vi "TDT-Initialize.vi"() -> (4 "Server IP Address":u32=4925, 6 "TCP Port":u16=4925, 14 "Data":T1={"TTankX"=refnum, "TDevAccX"=refnum, "LastTime"=0.0, "error"={"status"=FALSE, "code"=0, "source"=""}, "Block Name"="", "Circuit Tag"="", "Tank Name"="", "NumTicks"=0, "LastTick"=0.0, "Idle?"=FALSE, "Wait (ms)"=1000, "LastArtf"=0.0, "LastTosc"=0.0}, 15 "error out":errorcluster)   [LabVIEW 2015]
uses:
  TDT Interface Data.ctl
  <vilib>/Utility/config.llb/Read Key (String).vi
  <vilib>/Utility/config.llb/Read Key (I32).vi
  <vilib>/Utility/config.llb/Read Key (Boolean).vi
  <vilib>/Utility/config.llb/NI_LVConfig.lvlib
panel:
  in  "error in (no error)":errorcluster
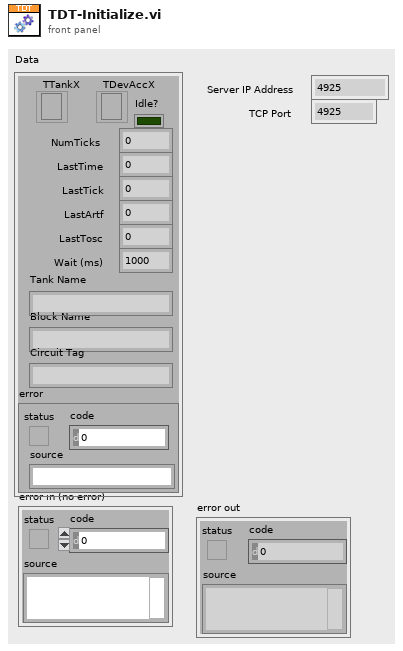
[diagram p1: front panel]
types:
  T1 = typedef "TDT Interface Data.ctl" = cluster{"TTankX":refnum<k7>, "TDevAccX":refnum<k7>, "LastTime":dbl, "error":errorcluster, "Block Name":string, "Circuit Tag":string, "Tank Name":string, "NumTicks":i32, "LastTick":dbl, "Idle?":bool, "Wait (ms)":u32, "LastArtf":dbl, "LastTosc":dbl}
  T2 = typedef "NI_LVConfig.lvlib/Config Data RefNum.ctl" = refnum<k1>
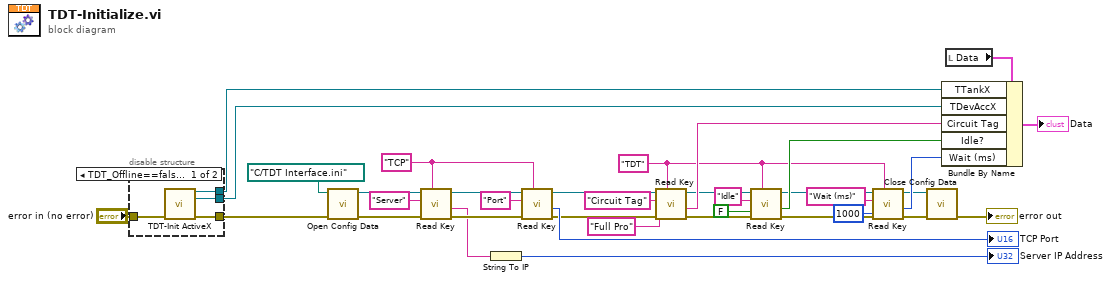
[diagram p0: block diagram]
diagram:
  w2 = "TDT" ("section")
  w29 = "TCP" ("section")
  n1 = disable-structure shown="TDT_Offline==false, Default" {
    disable-tunnel: "error in (no error)" -> [w40 _]
    disable-tunnel: [w39 _] -> w21
    disable-tunnel: [w38 _] -> w20
    disable-tunnel: [w37 _] -> w19
    frame condition #0 (active) {
      n2 = call "TDT-Init ActiveX.vi"("error in (no error)"=w40) -> ("TTANKXLib.TTankX"=w39:refnum<k7>, "TDEVACCXLib.TDevAccX"=w38:refnum<k7>, "error out"=w37:errorcluster)  [unwired: 12 in]
    }
    frame condition #1 {
    }
  }
  n3 = call <vilib>:"Open Config Data.vi"("error in (no error)"=w19, "configuration file path"=path "C:/TDT Interface.ini") -> ("error out"=w33:errorcluster, "refnum"=w34:T2)  [unwired: 7 in, 1 out]
  n4 = call-poly <vilib>:"Read Key.vi"("section"=w29, "error in (no error)"=w33, "key"="Server", "refnum"=w34) -> ("error out"=w31:errorcluster, "value"=w27:string, "refnum out"=w30:T2)  [unwired: 4 in, 1 out]
  n5 = String To IP(1:w27) -> (0:→"Server IP Address":u32)
  n6 = call-poly <vilib>:"Read Key.vi"("section"=w29, "error in (no error)"=w31, "key"="Port", "refnum"=w30) -> ("error out"=w17:errorcluster, "value"=→"TCP Port":i32, "refnum out"=w18:T2)  [unwired: 4 in, 1 out]
  n7 = call-poly <vilib>:"Read Key.vi"("section"=w2, "error in (no error)"=w17, "default value"="Full Pro", "key"="Circuit Tag", "refnum"=w18) -> ("error out"=w12:errorcluster, "value"=w14:string, "refnum out"=w11:T2)  [unwired: 3 in, 1 out]
  n8 = call-poly <vilib>:"Read Key.vi"("section"=w2, "error in (no error)"=w12, "default value"=FALSE, "key"="Idle", "refnum"=w11) -> ("error out"=w7:errorcluster, "value"=w9:bool, "refnum out"=w3:T2)  [unwired: 3 in, 1 out]
  n9 = call-poly <vilib>:"Read Key.vi"("section"=w2, "error in (no error)"=w7, "default value"=1000, "key"="Wait (ms)", "refnum"=w3) -> ("error out"=w6:errorcluster, "value"=w4:i32, "refnum out"=w1:T2)  [unwired: 3 in, 1 out]
  n10 = call <vilib>:"Close Config Data.vi"("error in (no error)"=w6, "refnum"=w1) -> ("error out"=→"error out":errorcluster)  [unwired: 8 in, 1 out]
  n11 = local read "Data"() -> (w22:T1)
  n12 = Bundle By Name(cluster=w22, "TTankX"=w21, "TDevAccX"=w20, "Circuit Tag"=w14, "Idle?"=w9, "Wait (ms)"=w4) -> (→"Data":T1)
